vi "4290_auto.vi"() -> ()   [LabVIEW 2010, in "4290_RingItUp.lvrbt"]
uses:
  4290_RingItUp.lvrbt
  <vilib>/FTC/FTC ControllerState.ctl
  <vilib>/FTC/FTC POVState.ctl
  <vilib>/NXT/Block Support/NXT_ButtonSelector.ctl
  <vilib>/NXT/Subs/LVHSConnector.ctl
  <vilib>/NXT/Block Support/NXT_InputPort.ctl
  <vilib>/NXT/NXTIO Xnodes/AddressXNode/NXTIOAddress.xnode
  <vilib>/NXT/Subs/MotorXNode.Servo Type.ctl
  <vilib>/NXT/Subs/MotorXNode.1Servo.ctl
  <vilib>/NXT/Subs/MotorXNode.DC Motor Type.ctl
  <vilib>/NXT/Subs/MotorXNode.2DCMotor.ctl
  <vilib>/NXT/NXTIO Xnodes/NXTIOXNode/NXTIO.xnode
  <vilib>/NXT/Subs/MotorXNode.1DCMotor.ctl
  <vilib>/NXT/Dual Mode Library/Display/drawText.vi
  <vilib>/NXT/Dual Mode Library/Display/clearDisplay.vi
  <vilib>/NXT/Dual Mode Library/Sensors/readNXTButton.vi
  <vilib>/NXT/Dual Mode Library/Waits/Wait_Num(msec).vi
  <vilib>/NXT/Dual Mode Library/Sensors/Touch_Pressed.vi
  <vilib>/NXT/Dual Mode Library/prims/inRangeAndCoerce/inRangeAndCoerce_float.vi
  <vilib>/NXT/Dual Mode Library/prims/inRangeAndCoerce/inRangeAndCoerce_int.vi
  <vilib>/NXT/Dual Mode Library/Display/drawNumber.vi
  <vilib>/NXT/NXTIO Xnodes/NXTIONodeSubVIs/TETRIX IO Move Servos.vi
  <vilib>/NXT/NXTIO Xnodes/NXTIONodeSubVIs/TETRIX IO Move DC Motors.vi
  5998_RingItUp/5998_RingItUp.lvrbt
panel:
  in  "step":u8=5
  in  "ClawPosition":u8=127
  in  "Direction":dbl
  out "Enabled":bool
  out "Controller State":T1={"Left X"=0, "Left Y"=0, "Right X"=0, "Right Y"=0, "Button Encoding 9-12"=0, "Button Encoding 1-8"=0, "POV"=-1} {"POV" items=["None"=-1, "POV Up"=0, "POV Up Right"=1, "POV Right"=2, "POV Down Right"=3, "POV Down"=4, "POV Down Left"=5, "POV Left"=6, "POV Up Left"=7]}
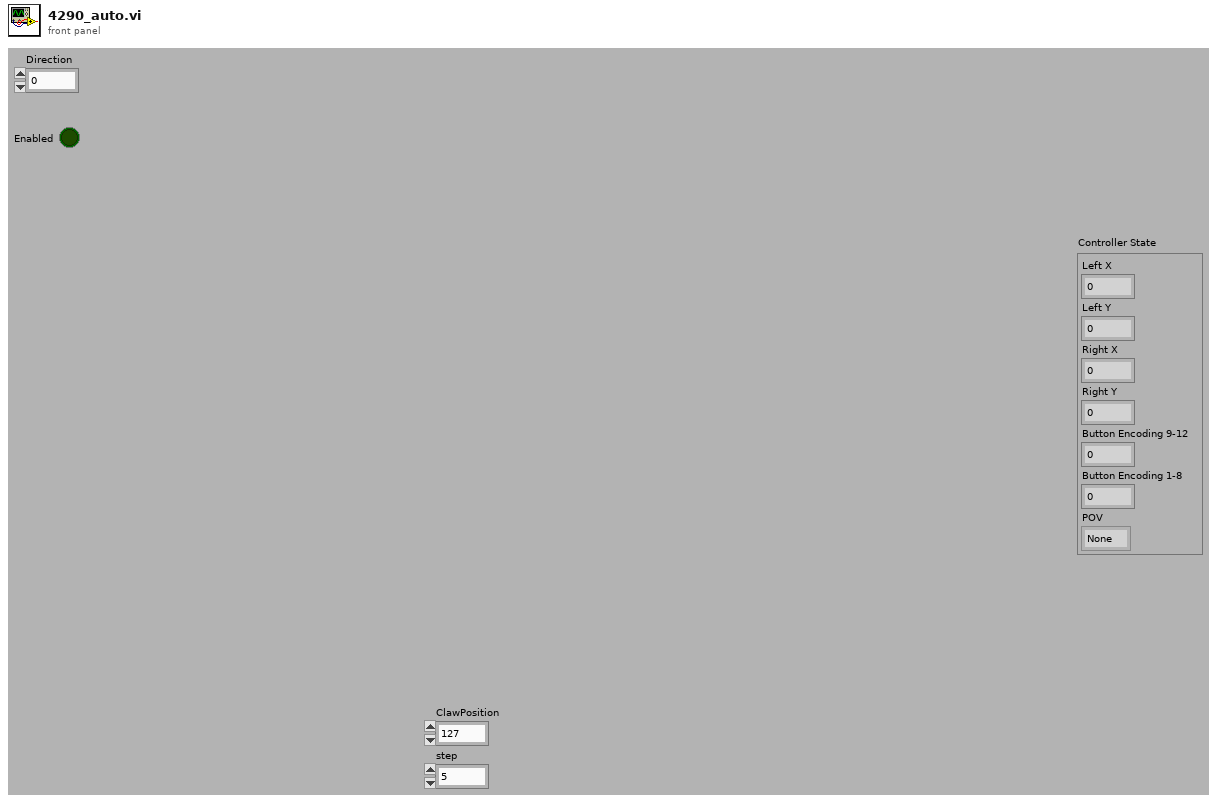
[diagram p1: front panel]
types:
  T1 = typedef "FTC ControllerState.ctl" = cluster{"Left X":i8, "Left Y":i8, "Right X":i8, "Right Y":i8, "Button Encoding 9-12":u8, "Button Encoding 1-8":u8, "POV":T2}
  T2 = typedef "FTC POVState.ctl" = i8
  T3 = typedef "NXT_ButtonSelector.ctl" = u16
  T4 = typedef "LVHSConnector.ctl" = cluster{"Hardware":string, "Flattened String":string}
  T5 = typedef "NXT_InputPort.ctl" = u8
  T6 = typedef "MotorXNode.Servo Type.ctl" = enum16{"Servo"}
  T7 = typedef "MotorXNode.DC Motor Type.ctl" = enum16{"DC Motor"}
  T8 = cluster{"DC Motor":T7, "Address":i16, "Address":i16}
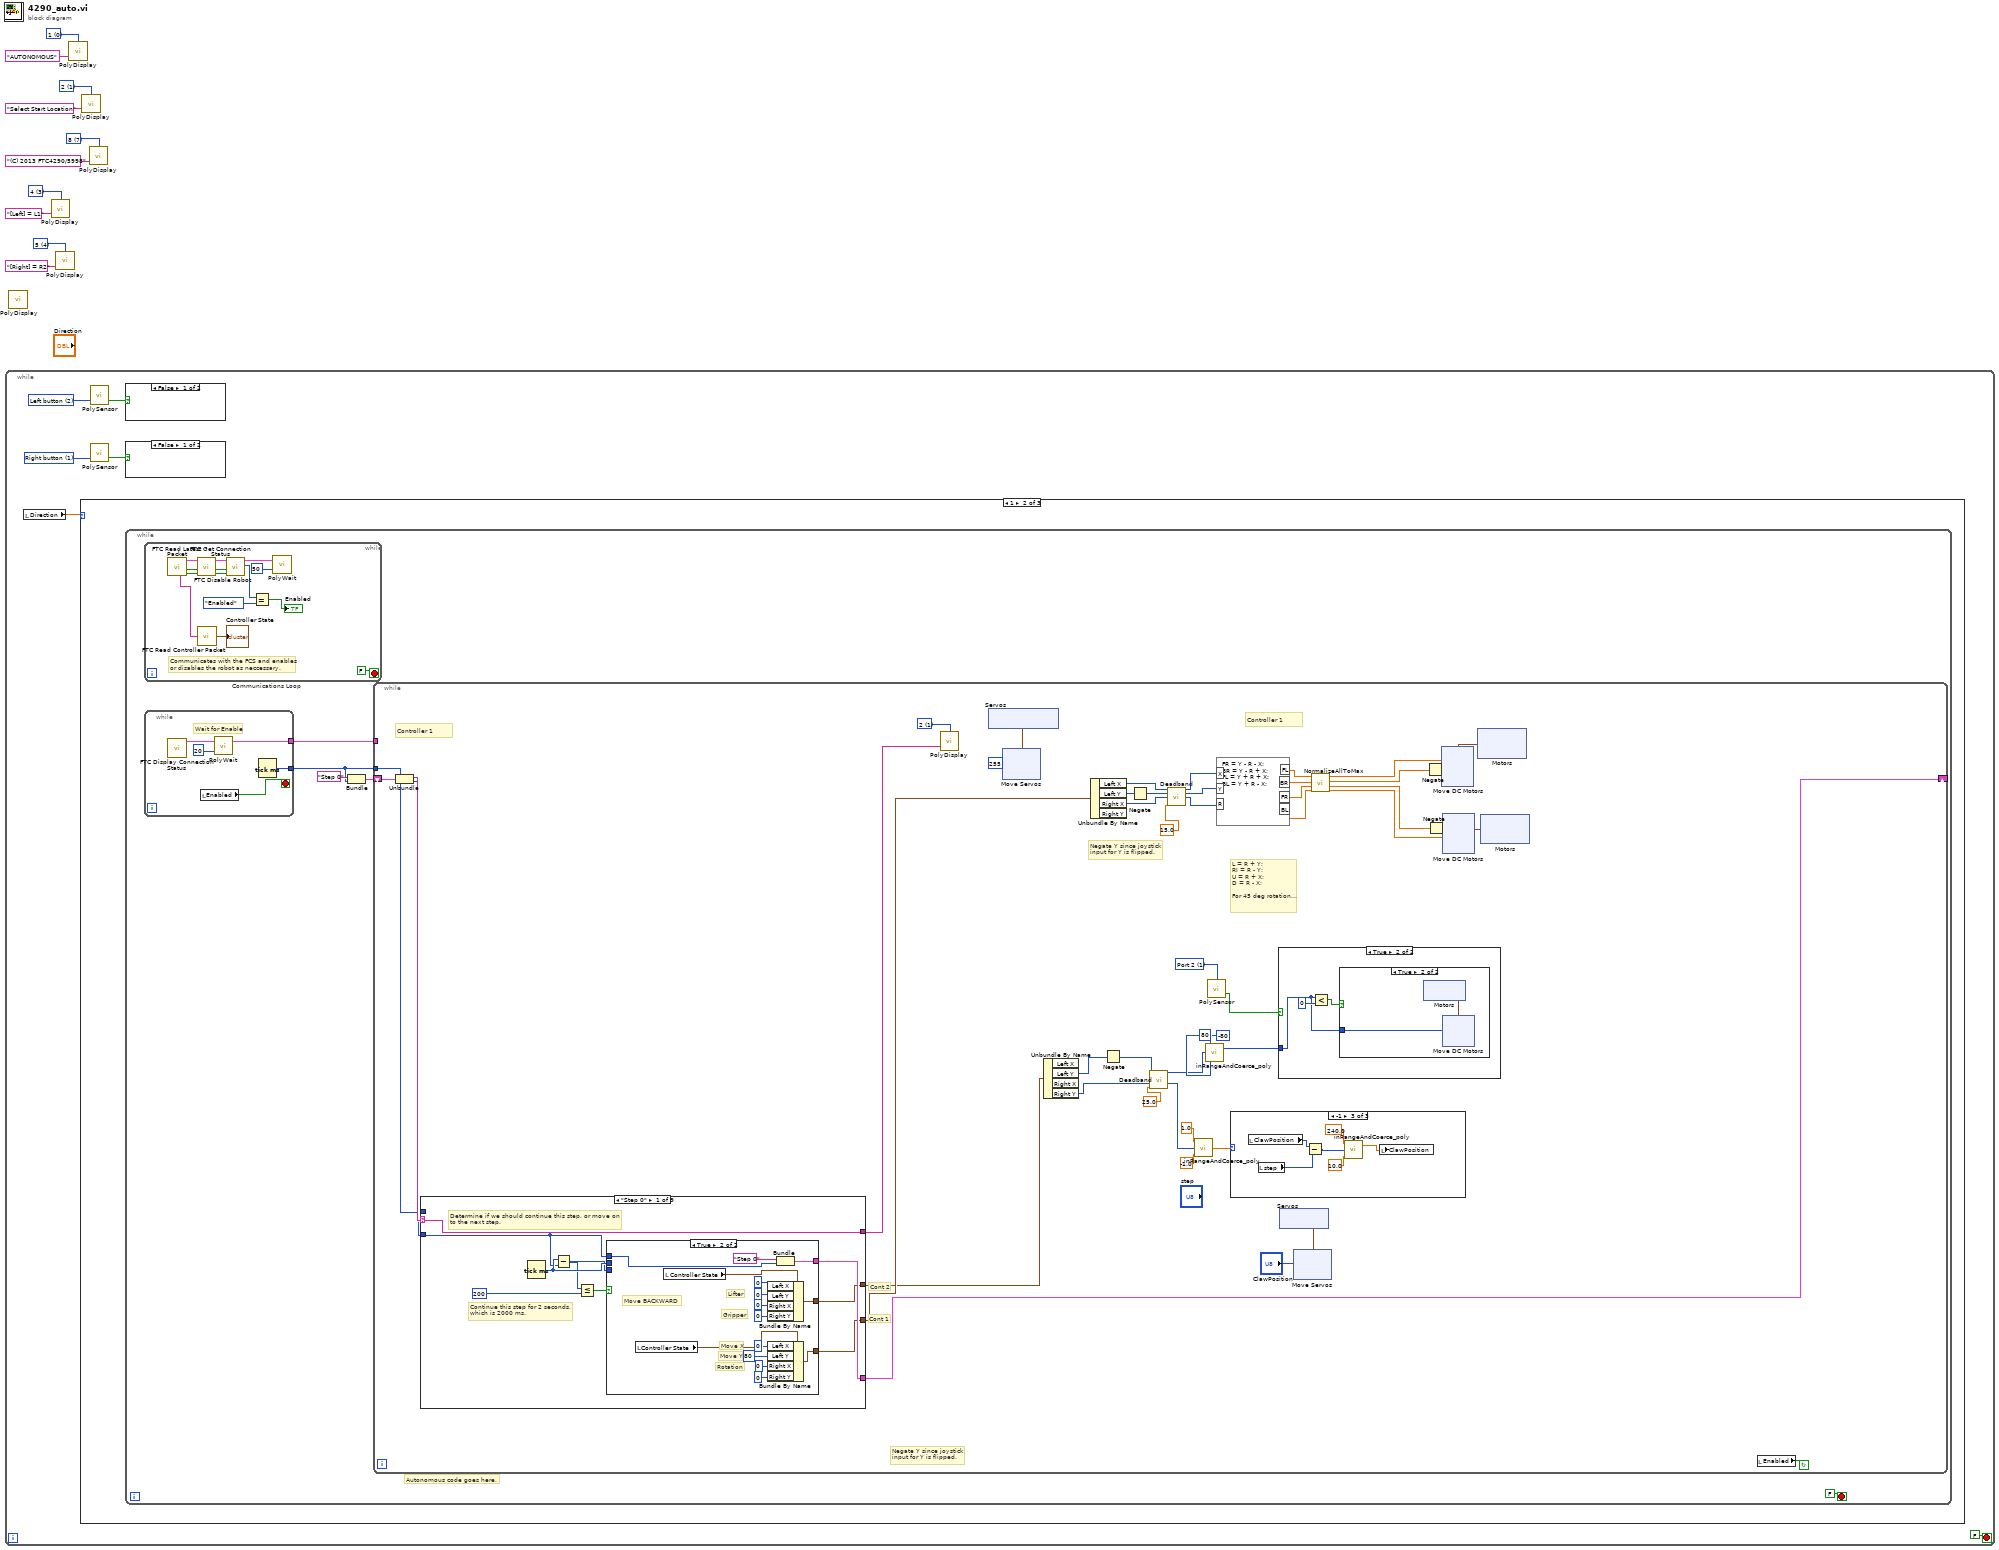
[diagram p0: block diagram]
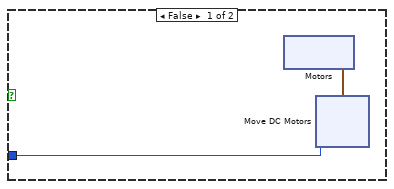
[diagram p3: hidden frame]
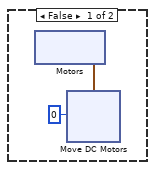
[diagram p4: hidden frame]
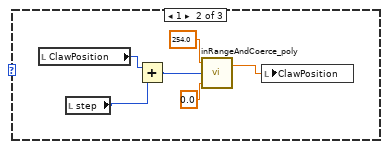
[diagram p6: hidden frame]
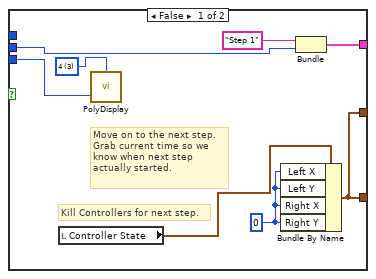
[diagram p7: hidden frame]
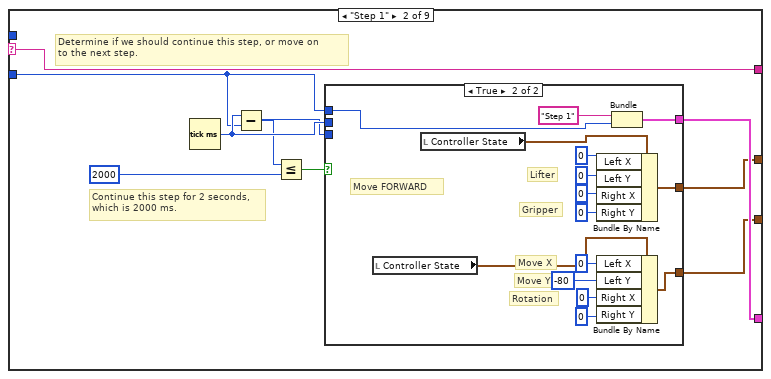
[diagram p8: hidden frame]
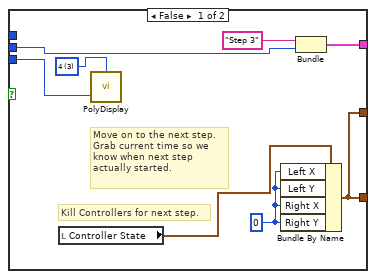
[diagram p9: hidden frame]
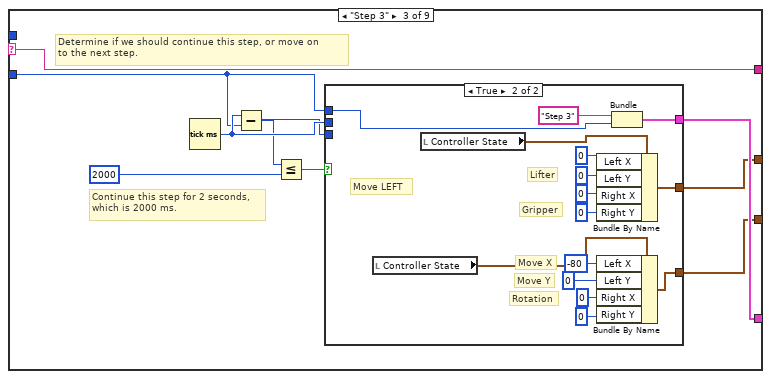
[diagram p10: hidden frame]
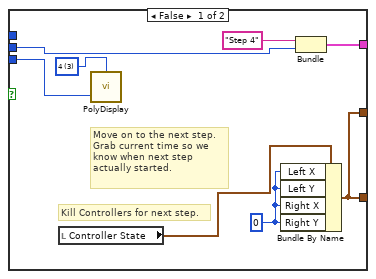
[diagram p11: hidden frame]
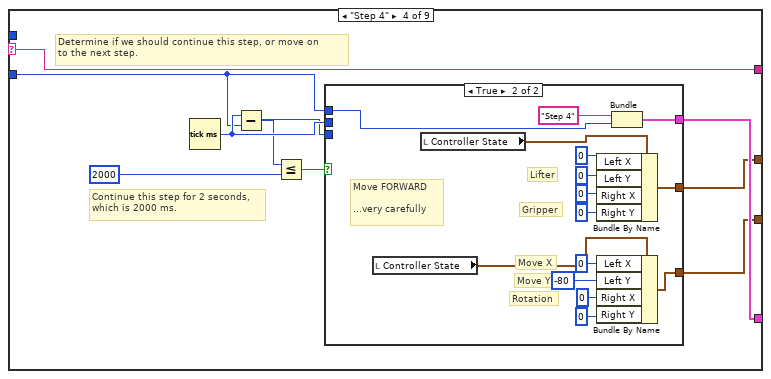
[diagram p12: hidden frame]
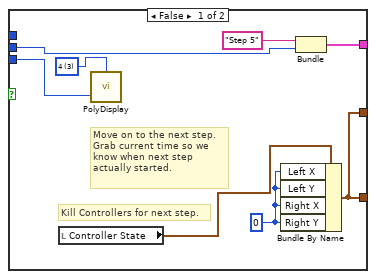
[diagram p13: hidden frame]
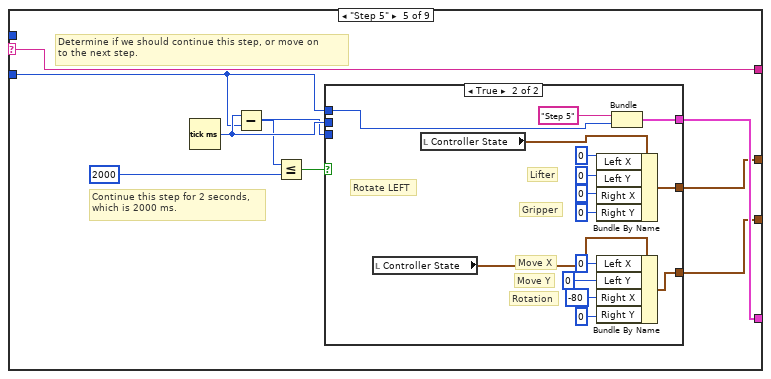
[diagram p14: hidden frame]
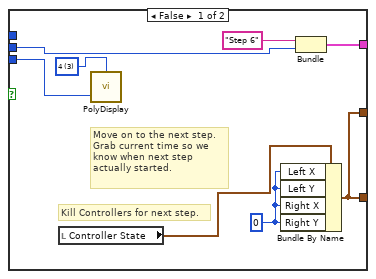
[diagram p15: hidden frame]
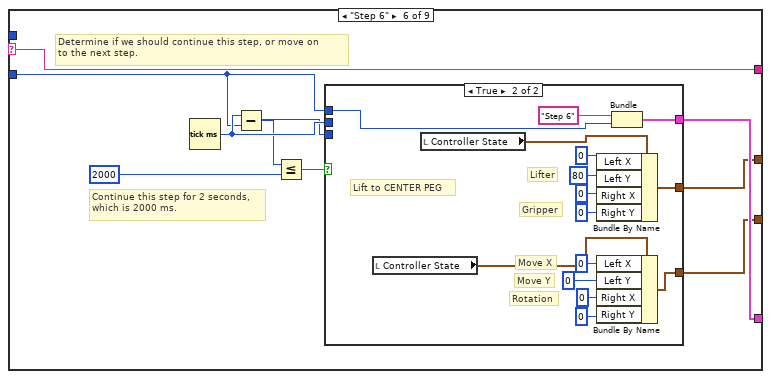
[diagram p16: hidden frame]
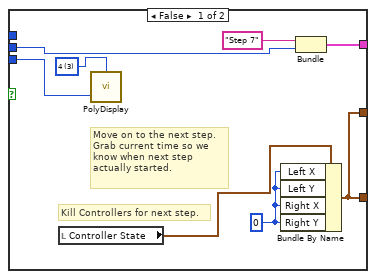
[diagram p17: hidden frame]
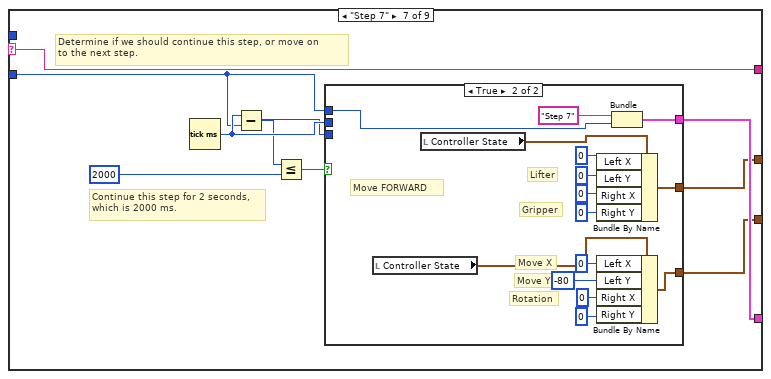
[diagram p18: hidden frame]
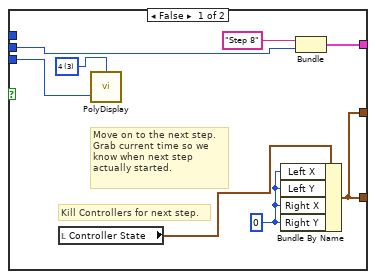
[diagram p19: hidden frame]
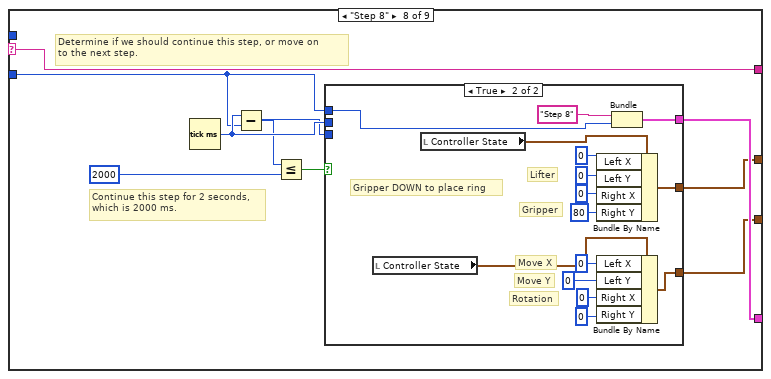
[diagram p20: hidden frame]
diagram:
  w2 = i16 7 items=["1", "2", "3", "4", "5", "6", "7", "8"] ("Line")
  w4 = i16 1 items=["1", "2", "3", "4", "5", "6", "7", "8"] ("Line")
  w6 = i16 4 items=["1", "2", "3", "4", "5", "6", "7", "8"] ("Line")
  w8 = i16 3 items=["1", "2", "3", "4", "5", "6", "7", "8"] ("Line")
  w10 = i16 0 items=["1", "2", "3", "4", "5", "6", "7", "8"] ("Line")
  n1 = while {
    stop <- FALSE stop-if-true
    w15 = T3 1 items=["Enter button"=3, "Left button"=2, "Right button"=1] ("Button (Enter button)")
    w16 = T3 2 items=["Enter button"=3, "Left button"=2, "Right button"=1] ("Button (Enter button)")
    n2 = local read "Direction"() -> (w11:dbl)
    n3 = case shown="1" w11 {
      frame 0, Default {
      }
      frame 1 {
        n4 = while {
          stop <- FALSE stop-if-true
          # "Autonomous code goes here."
          n5 = while "Communications Loop" {
            stop <- FALSE stop-if-true
            # "Communicates with the FCS and enables \nor disables the robot as neccessary."
            n6 = call <vilib>:"FTC Read Latest Packet.vi"() -> ("Packet Received?"=w444:bool, "Stopped?"=w443:bool, "NXT"=w446:T4, "Controller 1"=w434:string)  [unwired: 6 in, 2 out]
            n7 = call <vilib>:"FTC Get Connection Status.vi"("Packet Received?"=w444, "Stopped?"=w443, "NXT"=w446) -> ("Online?"=w435:bool, "Stopped?"=w436:bool, "NXT"=w445:T4)  [unwired: 5 in]
            n8 = call <vilib>:"FTC Read Controller Packet.vi"("Packet"=w434) -> ("Controller State"=→"Controller State":T1)  [unwired: 4 in]
            n9 = call <vilib>:"FTC Disable Robot.vi"("Online?"=w435, "Stopped?"=w436, "NXT"=w445) -> ("Enabled?"=w439:enum16{"Disabled", "Enabled"}, "NXT"=w441:T4)  [unwired: 3 in]
            n10 = Equal?(x=w439, y=enum16{"Disabled", "Enabled"}."Enabled") -> (x = y?=→"Enabled":bool)
            n11 = call-poly <vilib>:"PolyWait.vi"("Time (100 msec)"=u32 50 ("Time (msec)"), "NXT"=w441) -> ()  [unwired: 2 in, 1 out]
          }
          n12 = while {
            tunnel: [w431] -> w20
            tunnel: [w429] -> w17
            stop <- w428 stop-if-true
            # "Wait for Enable"
            n13 = call <vilib>:"FTC Display Connection Status.vi"() -> ("NXT"=w430:T4)  [unwired: 11 in]
            n14 = local read "Enabled"() -> (w428:bool)
            n15 = call-poly <vilib>:"PolyWait.vi"("Time (100 msec)"=u32 20 ("Time (msec)"), "NXT"=w430) -> ("NXT"=w431:T4)  [unwired: 2 in]
            n16 = Tick Count (ms)() -> (millisecond timer value=w429:u32)
          }
          n17 = Bundle("Step 0", "millisecond timer value"=w17) -> (w18:cluster{string, "millisecond timer value":u32})  [unwired: 1 in]
          n18 = while {
            tunnel: w20 -> [_]
            shift-right: [w66] -> _
            shift-left: w18 -> [w69]
            tunnel: w17 -> [w62]
            stop <- w65 continue-if-true
            w25 = T5 1 items=["Port 1", "Port 2", "Port 3", "Port 4"] ("Port (Port 1)")
            w64 = i16 1 items=["1", "2", "3", "4", "5", "6", "7", "8"] ("Line")
            # "L = R + Y;\nRI = R - Y;\nU = R + X;\nD = R - X;\n\nFor 45 deg rotation..."
            # "Negate Y since joystick\ninput for Y is flipped."
            # "Controller 1"
            # "Cont 1"
            # "Cont 2"
            # "Negate Y since joystick\ninput for Y is flipped."
            # "Controller 1"
            n19 = Unbundle(w69) -> (w68:string, "millisecond timer value"=w67:u32)
            n20 = case shown="\"Step 0\"" w68 {
              selector: w68 -> [w159 w191 w223 w255 w287 w319 w351 w383 w418]
              tunnel: [w166 w198 w230 w262 w294 w326 w358 w390 w423] -> w66
              tunnel: [w165 w197 w229 w261 w293 w325 w357 w389 w421] -> w39
              tunnel: w67 -> [w163 w195 w227 w259 w291 w323 w355 w387 _]
              tunnel: [w160 w192 w224 w256 w288 w320 w352 w384 w419] -> w22
              tunnel: [w159 w191 w223 w255 w287 w319 w351 w383 w418] -> w63
              tunnel: w62 -> [_ _ _ _ _ _ _ _ w415]
              frame "Step 0" {
                # "Continue this step for 2 seconds,\nwhich is 2000 ms."
                # "Determine if we should continue this step, or move on \nto the next step."
                n21 = Tick Count (ms)() -> (millisecond timer value=w164:u32)
                n22 = Subtract(x=w164, y=w163) -> (x-y=w158:u32)
                n23 = Less Or Equal?(x=w158, y=u32 200) -> (x <= y?=w161:bool)
                n24 = case shown="True" w161 {
                  tunnel: [w172 w184] -> w166
                  tunnel: [w169 w188] -> w165
                  tunnel: w164 -> [w174 _]
                  tunnel: w163 -> [_ w183]
                  tunnel: [w169 w186] -> w160
                  tunnel: w158 -> [w167 _]
                  frame False {
                    w168 = i16 3 items=["1", "2", "3", "4", "5", "6", "7", "8"] ("Line")
                    w170 = 0
                    # "Kill Controllers for next step."
                    # "Move on to the next step.\nGrab current time so we \nknow when next step \nactually started."
                    n25 = local read "Controller State"() -> (w171:T1)
                    n26 = call-poly <vilib>:"PolyDisplay.vi"("number"=w167, "Line"=w168) -> ()  [unwired: 2 in, 1 out]
                    n27 = Bundle By Name(cluster=w171, "Left X"=w170, "Left Y"=w170, "Right X"=w170, "Right Y"=w170) -> (w169:T1)
                    n28 = Bundle("Step 1", "millisecond timer value"=w174) -> (w172:cluster{string, "millisecond timer value":u32})  [unwired: 1 in]
                  }
                  frame True {
                    # "Gripper"
                    # "Lifter"
                    # "Rotation"
                    # "Move Y"
                    # "Move X"
                    # "Move BACKWARD"
                    n29 = local read "Controller State"() -> (w189:T1)
                    n30 = local read "Controller State"() -> (w187:T1)
                    n31 = Bundle By Name(cluster=w187, "Left X"=i8 0, "Left Y"=i8 0, "Right X"=i8 0, "Right Y"=i8 0) -> (w186:T1)
                    n32 = Bundle By Name(cluster=w189, "Left X"=i8 0, "Left Y"=i8 80, "Right X"=i8 0, "Right Y"=i8 0) -> (w188:T1)
                    n33 = Bundle("Step 0", "millisecond timer value"=w183) -> (w184:cluster{string, "millisecond timer value":u32})  [unwired: 1 in]
                  }
                }
              }
              frame "Step 1" {
                # "Continue this step for 2 seconds,\nwhich is 2000 ms."
                # "Determine if we should continue this step, or move on \nto the next step."
                n34 = Tick Count (ms)() -> (millisecond timer value=w196:u32)
                n35 = Subtract(x=w196, y=w195) -> (x-y=w190:u32)
                n36 = Less Or Equal?(x=w190, y=u32 2000) -> (x <= y?=w193:bool)
                n37 = case shown="True" w193 {
                  tunnel: [w204 w216] -> w198
                  tunnel: [w201 w220] -> w197
                  tunnel: w196 -> [w206 _]
                  tunnel: w195 -> [_ w215]
                  tunnel: [w201 w218] -> w192
                  tunnel: w190 -> [w199 _]
                  frame False {
                    w200 = i16 3 items=["1", "2", "3", "4", "5", "6", "7", "8"] ("Line")
                    w202 = 0
                    # "Kill Controllers for next step."
                    # "Move on to the next step.\nGrab current time so we \nknow when next step \nactually started."
                    n38 = local read "Controller State"() -> (w203:T1)
                    n39 = call-poly <vilib>:"PolyDisplay.vi"("number"=w199, "Line"=w200) -> ()  [unwired: 2 in, 1 out]
                    n40 = Bundle By Name(cluster=w203, "Left X"=w202, "Left Y"=w202, "Right X"=w202, "Right Y"=w202) -> (w201:T1)
                    n41 = Bundle("Step 3", "millisecond timer value"=w206) -> (w204:cluster{string, "millisecond timer value":u32})  [unwired: 1 in]
                  }
                  frame True {
                    # "Gripper"
                    # "Lifter"
                    # "Rotation"
                    # "Move Y"
                    # "Move X"
                    # "Move FORWARD"
                    n42 = local read "Controller State"() -> (w221:T1)
                    n43 = local read "Controller State"() -> (w219:T1)
                    n44 = Bundle By Name(cluster=w219, "Left X"=i8 0, "Left Y"=i8 0, "Right X"=i8 0, "Right Y"=i8 0) -> (w218:T1)
                    n45 = Bundle By Name(cluster=w221, "Left X"=i8 0, "Left Y"=i8 -80, "Right X"=i8 0, "Right Y"=i8 0) -> (w220:T1)
                    n46 = Bundle("Step 1", "millisecond timer value"=w215) -> (w216:cluster{string, "millisecond timer value":u32})  [unwired: 1 in]
                  }
                }
              }
              frame "Step 3" {
                # "Continue this step for 2 seconds,\nwhich is 2000 ms."
                # "Determine if we should continue this step, or move on \nto the next step."
                n47 = Tick Count (ms)() -> (millisecond timer value=w228:u32)
                n48 = Subtract(x=w228, y=w227) -> (x-y=w222:u32)
                n49 = Less Or Equal?(x=w222, y=u32 2000) -> (x <= y?=w225:bool)
                n50 = case shown="True" w225 {
                  tunnel: [w236 w248] -> w230
                  tunnel: [w233 w252] -> w229
                  tunnel: w228 -> [w238 _]
                  tunnel: w227 -> [_ w247]
                  tunnel: [w233 w250] -> w224
                  tunnel: w222 -> [w231 _]
                  frame False {
                    w232 = i16 3 items=["1", "2", "3", "4", "5", "6", "7", "8"] ("Line")
                    w234 = 0
                    # "Kill Controllers for next step."
                    # "Move on to the next step.\nGrab current time so we \nknow when next step \nactually started."
                    n51 = local read "Controller State"() -> (w235:T1)
                    n52 = call-poly <vilib>:"PolyDisplay.vi"("number"=w231, "Line"=w232) -> ()  [unwired: 2 in, 1 out]
                    n53 = Bundle By Name(cluster=w235, "Left X"=w234, "Left Y"=w234, "Right X"=w234, "Right Y"=w234) -> (w233:T1)
                    n54 = Bundle("Step 4", "millisecond timer value"=w238) -> (w236:cluster{string, "millisecond timer value":u32})  [unwired: 1 in]
                  }
                  frame True {
                    # "Gripper"
                    # "Lifter"
                    # "Rotation"
                    # "Move Y"
                    # "Move X"
                    # "Move LEFT"
                    n55 = local read "Controller State"() -> (w253:T1)
                    n56 = local read "Controller State"() -> (w251:T1)
                    n57 = Bundle By Name(cluster=w251, "Left X"=i8 0, "Left Y"=i8 0, "Right X"=i8 0, "Right Y"=i8 0) -> (w250:T1)
                    n58 = Bundle By Name(cluster=w253, "Left X"=i8 -80, "Left Y"=i8 0, "Right X"=i8 0, "Right Y"=i8 0) -> (w252:T1)
                    n59 = Bundle("Step 3", "millisecond timer value"=w247) -> (w248:cluster{string, "millisecond timer value":u32})  [unwired: 1 in]
                  }
                }
              }
              frame "Step 4" {
                # "Continue this step for 2 seconds,\nwhich is 2000 ms."
                # "Determine if we should continue this step, or move on \nto the next step."
                n60 = Tick Count (ms)() -> (millisecond timer value=w260:u32)
                n61 = Subtract(x=w260, y=w259) -> (x-y=w254:u32)
                n62 = Less Or Equal?(x=w254, y=u32 2000) -> (x <= y?=w257:bool)
                n63 = case shown="True" w257 {
                  tunnel: [w268 w280] -> w262
                  tunnel: [w265 w284] -> w261
                  tunnel: w260 -> [w270 _]
                  tunnel: w259 -> [_ w279]
                  tunnel: [w265 w282] -> w256
                  tunnel: w254 -> [w263 _]
                  frame False {
                    w264 = i16 3 items=["1", "2", "3", "4", "5", "6", "7", "8"] ("Line")
                    w266 = 0
                    # "Kill Controllers for next step."
                    # "Move on to the next step.\nGrab current time so we \nknow when next step \nactually started."
                    n64 = local read "Controller State"() -> (w267:T1)
                    n65 = call-poly <vilib>:"PolyDisplay.vi"("number"=w263, "Line"=w264) -> ()  [unwired: 2 in, 1 out]
                    n66 = Bundle By Name(cluster=w267, "Left X"=w266, "Left Y"=w266, "Right X"=w266, "Right Y"=w266) -> (w265:T1)
                    n67 = Bundle("Step 5", "millisecond timer value"=w270) -> (w268:cluster{string, "millisecond timer value":u32})  [unwired: 1 in]
                  }
                  frame True {
                    # "Gripper"
                    # "Lifter"
                    # "Rotation"
                    # "Move Y"
                    # "Move X"
                    # "Move FORWARD\n\n...very carefully"
                    n68 = local read "Controller State"() -> (w285:T1)
                    n69 = local read "Controller State"() -> (w283:T1)
                    n70 = Bundle By Name(cluster=w283, "Left X"=i8 0, "Left Y"=i8 0, "Right X"=i8 0, "Right Y"=i8 0) -> (w282:T1)
                    n71 = Bundle By Name(cluster=w285, "Left X"=i8 0, "Left Y"=i8 -80, "Right X"=i8 0, "Right Y"=i8 0) -> (w284:T1)
                    n72 = Bundle("Step 4", "millisecond timer value"=w279) -> (w280:cluster{string, "millisecond timer value":u32})  [unwired: 1 in]
                  }
                }
              }
              frame "Step 5" {
                # "Continue this step for 2 seconds,\nwhich is 2000 ms."
                # "Determine if we should continue this step, or move on \nto the next step."
                n73 = Tick Count (ms)() -> (millisecond timer value=w292:u32)
                n74 = Subtract(x=w292, y=w291) -> (x-y=w286:u32)
                n75 = Less Or Equal?(x=w286, y=u32 2000) -> (x <= y?=w289:bool)
                n76 = case shown="True" w289 {
                  tunnel: [w300 w312] -> w294
                  tunnel: [w297 w316] -> w293
                  tunnel: w292 -> [w302 _]
                  tunnel: w291 -> [_ w311]
                  tunnel: [w297 w314] -> w288
                  tunnel: w286 -> [w295 _]
                  frame False {
                    w296 = i16 3 items=["1", "2", "3", "4", "5", "6", "7", "8"] ("Line")
                    w298 = 0
                    # "Kill Controllers for next step."
                    # "Move on to the next step.\nGrab current time so we \nknow when next step \nactually started."
                    n77 = local read "Controller State"() -> (w299:T1)
                    n78 = call-poly <vilib>:"PolyDisplay.vi"("number"=w295, "Line"=w296) -> ()  [unwired: 2 in, 1 out]
                    n79 = Bundle By Name(cluster=w299, "Left X"=w298, "Left Y"=w298, "Right X"=w298, "Right Y"=w298) -> (w297:T1)
                    n80 = Bundle("Step 6", "millisecond timer value"=w302) -> (w300:cluster{string, "millisecond timer value":u32})  [unwired: 1 in]
                  }
                  frame True {
                    # "Gripper"
                    # "Lifter"
                    # "Rotation"
                    # "Move Y"
                    # "Move X"
                    # "Rotate LEFT"
                    n81 = local read "Controller State"() -> (w317:T1)
                    n82 = local read "Controller State"() -> (w315:T1)
                    n83 = Bundle By Name(cluster=w315, "Left X"=i8 0, "Left Y"=i8 0, "Right X"=i8 0, "Right Y"=i8 0) -> (w314:T1)
                    n84 = Bundle By Name(cluster=w317, "Left X"=i8 0, "Left Y"=i8 0, "Right X"=i8 -80, "Right Y"=i8 0) -> (w316:T1)
                    n85 = Bundle("Step 5", "millisecond timer value"=w311) -> (w312:cluster{string, "millisecond timer value":u32})  [unwired: 1 in]
                  }
                }
              }
              frame "Step 6" {
                # "Continue this step for 2 seconds,\nwhich is 2000 ms."
                # "Determine if we should continue this step, or move on \nto the next step."
                n86 = Tick Count (ms)() -> (millisecond timer value=w324:u32)
                n87 = Subtract(x=w324, y=w323) -> (x-y=w318:u32)
                n88 = Less Or Equal?(x=w318, y=u32 2000) -> (x <= y?=w321:bool)
                n89 = case shown="True" w321 {
                  tunnel: [w332 w344] -> w326
                  tunnel: [w329 w348] -> w325
                  tunnel: w324 -> [w334 _]
                  tunnel: w323 -> [_ w343]
                  tunnel: [w329 w346] -> w320
                  tunnel: w318 -> [w327 _]
                  frame False {
                    w328 = i16 3 items=["1", "2", "3", "4", "5", "6", "7", "8"] ("Line")
                    w330 = 0
                    # "Kill Controllers for next step."
                    # "Move on to the next step.\nGrab current time so we \nknow when next step \nactually started."
                    n90 = local read "Controller State"() -> (w331:T1)
                    n91 = call-poly <vilib>:"PolyDisplay.vi"("number"=w327, "Line"=w328) -> ()  [unwired: 2 in, 1 out]
                    n92 = Bundle By Name(cluster=w331, "Left X"=w330, "Left Y"=w330, "Right X"=w330, "Right Y"=w330) -> (w329:T1)
                    n93 = Bundle("Step 7", "millisecond timer value"=w334) -> (w332:cluster{string, "millisecond timer value":u32})  [unwired: 1 in]
                  }
                  frame True {
                    # "Gripper"
                    # "Lifter"
                    # "Rotation"
                    # "Move Y"
                    # "Move X"
                    # "Lift to CENTER PEG"
                    n94 = local read "Controller State"() -> (w349:T1)
                    n95 = local read "Controller State"() -> (w347:T1)
                    n96 = Bundle By Name(cluster=w347, "Left X"=i8 0, "Left Y"=i8 80, "Right X"=i8 0, "Right Y"=i8 0) -> (w346:T1)
                    n97 = Bundle By Name(cluster=w349, "Left X"=i8 0, "Left Y"=i8 0, "Right X"=i8 0, "Right Y"=i8 0) -> (w348:T1)
                    n98 = Bundle("Step 6", "millisecond timer value"=w343) -> (w344:cluster{string, "millisecond timer value":u32})  [unwired: 1 in]
                  }
                }
              }
              frame "Step 7" {
                # "Continue this step for 2 seconds,\nwhich is 2000 ms."
                # "Determine if we should continue this step, or move on \nto the next step."
                n99 = Tick Count (ms)() -> (millisecond timer value=w356:u32)
                n100 = Subtract(x=w356, y=w355) -> (x-y=w350:u32)
                n101 = Less Or Equal?(x=w350, y=u32 2000) -> (x <= y?=w353:bool)
                n102 = case shown="True" w353 {
                  tunnel: [w364 w376] -> w358
                  tunnel: [w361 w380] -> w357
                  tunnel: w356 -> [w366 _]
                  tunnel: w355 -> [_ w375]
                  tunnel: [w361 w378] -> w352
                  tunnel: w350 -> [w359 _]
                  frame False {
                    w360 = i16 3 items=["1", "2", "3", "4", "5", "6", "7", "8"] ("Line")
                    w362 = 0
                    # "Kill Controllers for next step."
                    # "Move on to the next step.\nGrab current time so we \nknow when next step \nactually started."
                    n103 = local read "Controller State"() -> (w363:T1)
                    n104 = call-poly <vilib>:"PolyDisplay.vi"("number"=w359, "Line"=w360) -> ()  [unwired: 2 in, 1 out]
                    n105 = Bundle By Name(cluster=w363, "Left X"=w362, "Left Y"=w362, "Right X"=w362, "Right Y"=w362) -> (w361:T1)
                    n106 = Bundle("Step 8", "millisecond timer value"=w366) -> (w364:cluster{string, "millisecond timer value":u32})  [unwired: 1 in]
                  }
                  frame True {
                    # "Gripper"
                    # "Lifter"
                    # "Rotation"
                    # "Move Y"
                    # "Move X"
                    # "Move FORWARD"
                    n107 = local read "Controller State"() -> (w381:T1)
                    n108 = local read "Controller State"() -> (w379:T1)
                    n109 = Bundle By Name(cluster=w379, "Left X"=i8 0, "Left Y"=i8 0, "Right X"=i8 0, "Right Y"=i8 0) -> (w378:T1)
                    n110 = Bundle By Name(cluster=w381, "Left X"=i8 0, "Left Y"=i8 -80, "Right X"=i8 0, "Right Y"=i8 0) -> (w380:T1)
                    n111 = Bundle("Step 7", "millisecond timer value"=w375) -> (w376:cluster{string, "millisecond timer value":u32})  [unwired: 1 in]
                  }
                }
              }
              frame "Step 8" {
                # "Continue this step for 2 seconds,\nwhich is 2000 ms."
                # "Determine if we should continue this step, or move on \nto the next step."
                n112 = Tick Count (ms)() -> (millisecond timer value=w388:u32)
                n113 = Subtract(x=w388, y=w387) -> (x-y=w382:u32)
                n114 = Less Or Equal?(x=w382, y=u32 2000) -> (x <= y?=w385:bool)
                n115 = case shown="True" w385 {
                  tunnel: [w396 w408] -> w390
                  tunnel: [w393 w412] -> w389
                  tunnel: w388 -> [w398 _]
                  tunnel: w387 -> [_ w407]
                  tunnel: [w393 w410] -> w384
                  tunnel: w382 -> [w391 _]
                  frame False {
                    w392 = i16 3 items=["1", "2", "3", "4", "5", "6", "7", "8"] ("Line")
                    w394 = 0
                    # "Kill Controllers for next step."
                    # "Move on to the next step.\nGrab current time so we \nknow when next step \nactually started."
                    n116 = local read "Controller State"() -> (w395:T1)
                    n117 = call-poly <vilib>:"PolyDisplay.vi"("number"=w391, "Line"=w392) -> ()  [unwired: 2 in, 1 out]
                    n118 = Bundle By Name(cluster=w395, "Left X"=w394, "Left Y"=w394, "Right X"=w394, "Right Y"=w394) -> (w393:T1)
                    n119 = Bundle("STOP", "millisecond timer value"=w398) -> (w396:cluster{string, "millisecond timer value":u32})  [unwired: 1 in]
                  }
                  frame True {
                    # "Gripper"
                    # "Lifter"
                    # "Rotation"
                    # "Move Y"
                    # "Move X"
                    # "Gripper DOWN to place ring"
                    n120 = local read "Controller State"() -> (w413:T1)
                    n121 = local read "Controller State"() -> (w411:T1)
                    n122 = Bundle By Name(cluster=w411, "Left X"=i8 0, "Left Y"=i8 0, "Right X"=i8 0, "Right Y"=i8 80) -> (w410:T1)
                    n123 = Bundle By Name(cluster=w413, "Left X"=i8 0, "Left Y"=i8 0, "Right X"=i8 0, "Right Y"=i8 0) -> (w412:T1)
                    n124 = Bundle("Step 8", "millisecond timer value"=w407) -> (w408:cluster{string, "millisecond timer value":u32})  [unwired: 1 in]
                  }
                }
              }
              frame "STOP", Default {
                w417 = i16 2 items=["1", "2", "3", "4", "5", "6", "7", "8"] ("Line")
                w425 = 0
                w420 = 0
                # "KILL ROBOT"
                n125 = Tick Count (ms)() -> (millisecond timer value=w416:u32)
                n126 = Subtract(x=w416, y=w415) -> (x-y=w414:u32)
                n127 = call-poly <vilib>:"PolyDisplay.vi"("number"=w414, "Line"=w417) -> ()  [unwired: 2 in, 1 out]
                n128 = local read "Controller State"() -> (w426:T1)
                n129 = local read "Controller State"() -> (w427:T1)
                n130 = Bundle By Name(cluster=w426, "Left X"=w425, "Left Y"=w425, "Right X"=w425, "Right Y"=w425) -> (w419:T1)
                n131 = Bundle By Name(cluster=w427, "Left X"=w420, "Left Y"=w420, "Right X"=w420, "Right Y"=w420) -> (w421:T1)
                n132 = Bundle("STOP", 0) -> (w423:cluster{string, i32})  [unwired: 1 in]
              }
            }
            n133 = call-poly <vilib>:"PolyDisplay.vi"("Text"=w63, "Line"=w64) -> ()  [unwired: 2 in, 1 out]
            n134 = xnode "Servos"() -> ("Servo"=w61:cluster{"Servo":T6, "Address":i16})
            n135 = xnode "Move Servos"("Position 1"=u8 255, "Servos"=w61) -> ()  [unwired: 1 in, 1 out]
            n136 = Unbundle By Name(w22) -> ("Left Y"=w38:i8, "Right Y"=w37:i8)  [unwired: 2 out]
            n137 = Unbundle By Name(w39) -> ("Left X"=w59:i8, "Left Y"=w58:i8, "Right X"=w57:i8)  [unwired: 1 out]
            n138 = Negate(x=w38) -> (-x=w26:i8)
            n139 = Negate(x=w58) -> (-x=w50:i8)
            n140 = call "Deadband.vi"("A"=w26, "D"=w37, "Deadband"=25.0) -> ("A 2"=w33:i32, "D2"=w28:i32)  [unwired: 9 in, 2 out]
            n141 = call "Deadband.vi"("A"=w59, "B"=w50, "C"=w57, "Deadband"=15.0) -> ("A 2"=w55:i32, "B 2"=w54:i32, "C2"=w53:i32)  [unwired: 8 in, 1 out]
            n142 = call-poly <vilib>:"inRangeAndCoerce_poly.vi"("lower limit"=-1.0, "x"=w28, "upper limit"=1.0) -> ("coerced(x)"=w31:dbl)  [unwired: 1 out]
            n143 = call-poly <vilib>:"inRangeAndCoerce_poly.vi"("lower limit"=-80, "x"=w33, "upper limit"=80) -> ("coerced(x)"=w23:i32)  [unwired: 1 out]
            n144 = call-poly <vilib>:"PolySensor.vi"("Port (Port 1)"=w25) -> ("Yes / No"=w24:bool)  [unwired: 2 in, 1 out]
            n145 = formula code="FR = Y - R - X;\nBR = Y - R + X;\nFL = Y + R + X;\nBL = Y + R - X;"("X"=w55, "Y"=w54, "R"=w53) -> ("FR"=w48:dbl, "FL"=w46:dbl, "BR"=w47:dbl, "BL"=w49:dbl)
            n146 = case shown="-1" w31 {
              frame 0, Default {
              }
              frame 1 {
                n147 = local read "ClawPosition"() -> (w112:u8)
                n148 = local read "step"() -> (w107:u8)
                n149 = Add(x=w112, y=w107) -> (x+y=w109:u8)
                n150 = call-poly <vilib>:"inRangeAndCoerce_poly.vi"("lower limit"=0.0, "x"=w109, "upper limit"=254.0) -> ("coerced(x)"=w108:dbl)  [unwired: 1 out]
                n151 = local write "ClawPosition"(w108) -> ()
              }
              frame -1 {
                n152 = local read "ClawPosition"() -> (w118:u8)
                n153 = local read "step"() -> (w114:u8)
                n154 = Subtract(x=w118, y=w114) -> (x-y=w115:u8)
                n155 = call-poly <vilib>:"inRangeAndCoerce_poly.vi"("lower limit"=10.0, "x"=w115, "upper limit"=240.0) -> ("coerced(x)"=w113:dbl)  [unwired: 1 out]
                n156 = local write "ClawPosition"(w113) -> ()
              }
            }
            n157 = case shown="True" w24 {
              tunnel: w23 -> [w70 w81]
              frame False {
                n158 = xnode "Motors"() -> ("DC Motor"=w71:cluster{"DC Motor":T7, "Address":i16})
                n159 = xnode ("Move DC Motors")("Power/Speed 1"=w70, "Motors"=w71) -> ()  [unwired: 1 in, 1 out]
              }
              frame True {
                n160 = Less?(x=w81, y=0) -> (x < y?=w82:bool)
                n161 = case shown="True" w82 {
                  tunnel: w81 -> [_ w95]
                  frame False {
                    n162 = xnode "Motors"() -> ("DC Motor"=w85:cluster{"DC Motor":T7, "Address":i16})
                    n163 = xnode ("Move DC Motors")("Power/Speed 1"=i8 0, "Motors"=w85) -> ()  [unwired: 1 in, 1 out]
                  }
                  frame True {
                    n164 = xnode "Motors"() -> ("DC Motor"=w96:cluster{"DC Motor":T7, "Address":i16})
                    n165 = xnode ("Move DC Motors")("Power/Speed 1"=w95, "Motors"=w96) -> ()  [unwired: 1 in, 1 out]
                  }
                }
              }
            }
            n166 = xnode "Servos"() -> ("Servo"=w27:cluster{"Servo":T6, "Address":i16})
            n167 = xnode "Move Servos"("Position 1"="ClawPosition", "Servos"=w27) -> ()  [unwired: 1 in, 1 out]
            n168 = call "NormalizeAllToMax.vi"("BL"=w49, "FR"=w48, "FL"=w47, "BR"=w46) -> ("Normalized BL"=w51:dbl, "Normalized FR"=w44:dbl, "Normalized FL"=w52:dbl, "Normalized BR"=w45:dbl)
            n169 = Negate(x=w52) -> (-x=w41:dbl)
            n170 = Negate(x=w44) -> (-x=w40:dbl)
            n171 = xnode "Motors"() -> ("DC Motor"=w43:T8)
            n172 = xnode ("Move DC Motors")("Power/Speed 2"=w41, "Power/Speed 1"=w45, "Motors"=w43) -> ()  [unwired: 1 in, 1 out]
            n173 = xnode "Motors"() -> ("DC Motor"=w42:T8)
            n174 = xnode ("Move DC Motors")("Power/Speed 2"=w51, "Power/Speed 1"=w40, "Motors"=w42) -> ()  [unwired: 1 in, 1 out]
            n175 = local read "Enabled"() -> (w65:bool)
          }
        }
      }
      frame 2 {
      }
    }
    n176 = call-poly <vilib>:"PolySensor.vi"("Button (Enter button)"=w16) -> ("Yes/No"=w13:bool)  [unwired: 2 in, 1 out]
    n177 = call-poly <vilib>:"PolySensor.vi"("Button (Enter button)"=w15) -> ("Yes/No"=w14:bool)  [unwired: 2 in, 1 out]
    n178 = case shown="False" w13 {
      frame False {
      }
      frame True {
        n179 = local write "Direction"(1.0 ("Direction")) -> ()
      }
    }
    n180 = case shown="False" w14 {
      frame False {
      }
      frame True {
        n181 = local write "Direction"(2.0 ("Direction")) -> ()
      }
    }
  }
  n182 = call-poly <vilib>:"PolyDisplay.vi"() -> ()  [unwired: 4 in, 1 out]
  n183 = call-poly <vilib>:"PolyDisplay.vi"("Text"="[Left] = L1", "Line"=w8) -> ()  [unwired: 2 in, 1 out]
  n184 = call-poly <vilib>:"PolyDisplay.vi"("Text"="[Right] = R2", "Line"=w6) -> ()  [unwired: 2 in, 1 out]
  n185 = call-poly <vilib>:"PolyDisplay.vi"("Text"="AUTONOMOUS", "Line"=w10) -> ()  [unwired: 2 in, 1 out]
  n186 = call-poly <vilib>:"PolyDisplay.vi"("Text"="Select Start Location", "Line"=w4) -> ()  [unwired: 2 in, 1 out]
  n187 = call-poly <vilib>:"PolyDisplay.vi"("Text"="(C) 2013 FTC4290/5998", "Line"=w2) -> ()  [unwired: 2 in, 1 out]
